vi "Find Worksheet.vi"(8 "error in":errorcluster, 10 "Sheet Name":string, 11 "SpreadsheetDocument":refnum<k24>) -> (0 "error out":errorcluster, 1 "Worksheet":refnum<k24>, 2 "WorkbookPart":refnum<k24>, 3 "SpreadsheetDocument out":refnum<k24>)   [LabVIEW 2021, in "Open Xml.lvlib"]
uses:
  Open Xml.lvlib
  D:/git/Open-Xml-LabVIEW/Source/DocumentFormat.OpenXml.dll
  DocumentFormat.OpenXml.dll
  D:/git/Open-Xml-LabVIEW/Source/DocumentFormat.OpenXml.Framework.dll
  DocumentFormat.OpenXml.Framework.dll
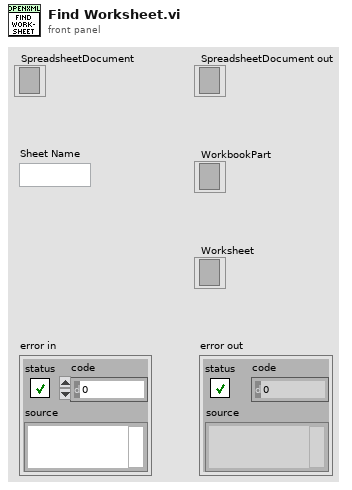
[diagram p1: front panel]
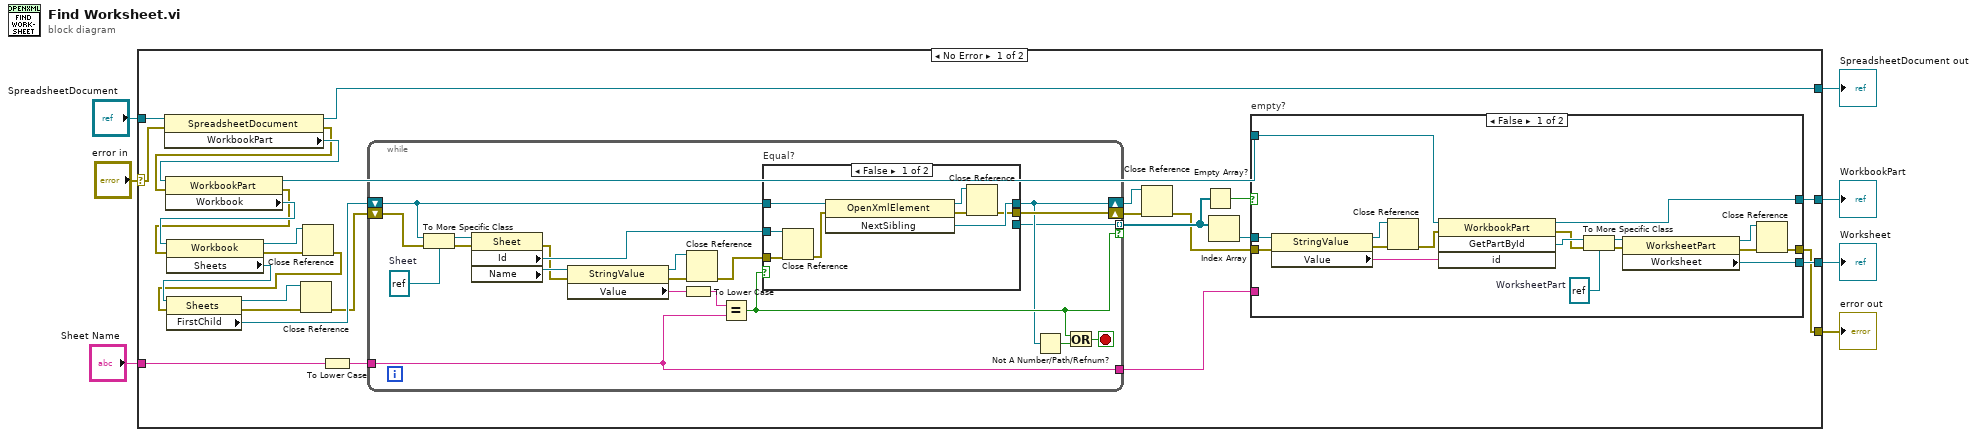
[diagram p0: block diagram]
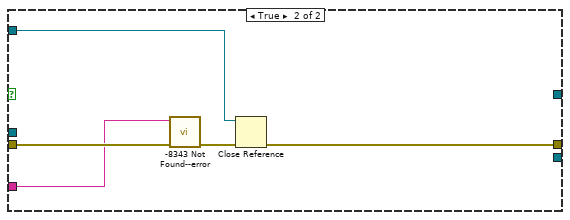
[diagram p3: hidden frame]
diagram:
  n1 = case shown="No Error" "error in" {
    selector: "error in" -> [w32 w89]
    tunnel: [w22 _] -> w6
    tunnel: [w21 w89] -> w5
    tunnel: [w20 _] -> w4
    tunnel: "Sheet Name" -> [w18 _]
    tunnel: "SpreadsheetDocument" -> [w10 _]
    tunnel: [w9 _] -> w1
    frame No Error {
      n2 = property class="SpreadsheetDocument"(reference=w10, error in=w32) -> (reference out=w9:refnum<k24>, error out=w31:errorcluster, "WorkbookPart"=w35:refnum<k24>)
      n3 = property class="WorkbookPart"(reference=w35, error in=w31) -> (reference out=w23:refnum<k24>, error out=w30:errorcluster, "Workbook"=w34:refnum<k24>)
      n4 = property class="Workbook"(reference=w34, error in=w30) -> (reference out=w13:refnum<k24>, error out=w29:errorcluster, "Sheets"=w33:refnum<k24>)
      n5 = Close Reference(reference=w13, error in (no error)=w29) -> (error out=w8:errorcluster)
      n6 = property class="Sheets"(reference=w33, error in=w8) -> (reference out=w11:refnum<k24>, error out=w26:errorcluster, "FirstChild"=w28:refnum<k24>)
      n7 = Close Reference(reference=w11, error in (no error)=w26) -> (error out=w12:errorcluster)
      n8 = To Lower Case(string=w18) -> (all lower case string=w27:string)
      n9 = while {
        tunnel: [w37] -> w25 mode=indexing if=w47
        tunnel: w27 -> [w41]
        shift-right: [w42] -> w14
        shift-left: w28 -> [w48]
        shift-right: [w45] -> w19
        shift-left: w12 -> [w49]
        tunnel: [w41] -> w17
        stop <- w44 stop-if-true
        w55 = refnum<k24> refnum  # Sheet
        n10 = To More Specific Class(target class=w55, reference=w48, error in=w49) -> (specific class reference=w53:refnum<k24>, error out=w54:errorcluster)
        n11 = property class="Sheet"(reference=w53, error in=w54) -> (error out=w36:errorcluster, "Id"=w38:refnum<k24>, "Name"=w52:refnum<k24>)  [unwired: 1 out]
        n12 = property class="StringValue"(reference=w52, error in=w36) -> (reference out=w39:refnum<k24>, error out=w46:errorcluster, "Value"=w51:string)
        n13 = To Lower Case(string=w51) -> (all lower case string=w50:string)
        n14 = Close Reference(reference=w39, error in (no error)=w46) -> (error out=w40:errorcluster)
        n15 = Equal?(x=w50, y=w41) -> (x = y?=w47:bool)
        n16 = case "Equal?" shown="False" w47 {
          tunnel: w48 -> [w63 w66]
          tunnel: [w62 w66] -> w42
          tunnel: w40 -> [w59 w65]
          tunnel: [w57 w65] -> w45
          tunnel: w38 -> [w60 w64]
          tunnel: [_ w64] -> w37
          frame False {
            n17 = Close Reference(reference=w60, error in (no error)=w59) -> (error out=w58:errorcluster)
            n18 = invoke class="OpenXmlElement" method="NextSibling"(reference=w63, error in=w58) -> (reference out=w56:refnum<k24>, error out=w61:errorcluster, "NextSibling"=w62:refnum<k24>)  [unwired: 1 in]
            n19 = Close Reference(reference=w56, error in (no error)=w61) -> (error out=w57:errorcluster)
          }
          frame True {
          }
        }
        n20 = Not A Number/Path/Refnum?(number/path/refnum=w42) -> (NaN/Path/Refnum?=w43:bool)
        n21 = Or(x=w47, y=w43) -> (x .or. y?=w44:bool)
      }
      n22 = Close Reference(reference=w14, error in (no error)=w19) -> (error out=w15:errorcluster)
      n23 = Empty Array?(array=w25) -> (empty?=w16:bool)
      n24 = Index Array(array=w25) -> (element=w24:refnum<k24>)  [unwired: 1 in]
      n25 = case "empty?" shown="False" w16 {
        tunnel: w24 -> [w83 _]
        tunnel: w15 -> [w82 w88]
        tunnel: w23 -> [w81 w84]
        tunnel: [w73 _] -> w22
        tunnel: [w70 w85] -> w21
        tunnel: [w71 _] -> w20
        tunnel: w17 -> [_ w86]
        frame False {
          w77 = refnum<k24> refnum  # WorksheetPart
          n26 = property class="StringValue"(reference=w83, error in=w82) -> (reference out=w67:refnum<k24>, error out=w79:errorcluster, "Value"=w80:string)
          n27 = Close Reference(reference=w67, error in (no error)=w79) -> (error out=w68:errorcluster)
          n28 = invoke class="WorkbookPart" method="GetPartById"(reference=w81, error in=w68, "id"=w80) -> (reference out=w71:refnum<k24>, error out=w76:errorcluster, "GetPartById"=w78:refnum<k24>)  [unwired: 1 in, 1 out]
          n29 = To More Specific Class(target class=w77, reference=w78, error in=w76) -> (specific class reference=w75:refnum<k24>, error out=w74:errorcluster)
          n30 = property class="WorksheetPart"(reference=w75, error in=w74) -> (reference out=w69:refnum<k24>, error out=w72:errorcluster, "Worksheet"=w73:refnum<k24>)
          n31 = Close Reference(reference=w69, error in (no error)=w72) -> (error out=w70:errorcluster)
        }
        frame True {
          n32 = call "-8343 Not Found--error.vi"("error in (no error)"=w88, "Item"=w86) -> ("error out"=w87:errorcluster)  [unwired: 9 in]
          n33 = Close Reference(reference=w84, error in (no error)=w87) -> (error out=w85:errorcluster)
        }
      }
    }
    frame Error {
    }
  }
  "error out" <- w5
  "Worksheet" <- w6
  "WorkbookPart" <- w4
  "SpreadsheetDocument out" <- w1
